vi "delete_element(array).vi"(8 "error in (no error)":errorcluster, 11 "data store (in)":cluster{"name":string, "address":string}[](array[cluster])) -> (0 "error out":errorcluster, 1 "deleted element":cluster{"name":string, "address":string}, 2 "element found ?":bool, 3 "data store (out)":cluster{"name":string, "address":string}[](array[cluster]))   [LabVIEW 2018]
panel:
  in  "name":string
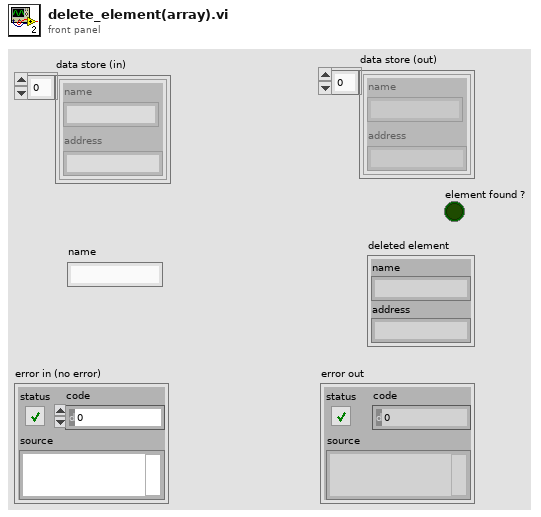
[diagram p1: front panel]
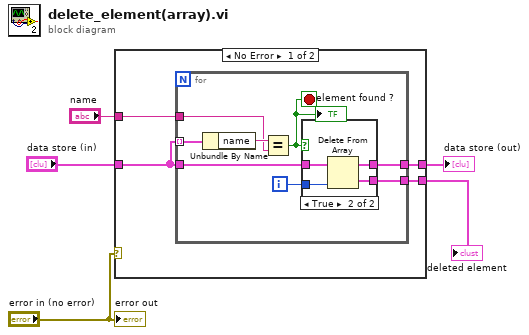
[diagram p0: block diagram]
diagram:
  n1 = case shown="No Error" "error in (no error)" {
    tunnel: "data store (in)" -> [w8 w23]
    tunnel: "name" -> [w9 _]
    tunnel: [w7 w23] -> w2
    tunnel: [w6 _] -> w1
    frame No Error {
      n2 = for {
        tunnel: w8 -> [w17] mode=indexing
        tunnel: w9 -> [w15]
        tunnel: w8 -> [w13]
        tunnel: [w12] -> w7
        tunnel: [w10] -> w6
        i -> [w14]
        stop <- w11 stop-if-true
        n3 = Unbundle By Name(w17) -> ("name"=w16:string)
        n4 = Equal?(x=w16, y=w15) -> (x = y?=w11:bool)
        "element found ?" <- w11
        n5 = case shown="True" w11 {
          tunnel: w14 -> [_ w22]
          tunnel: w13 -> [w18 w21]
          tunnel: [w18 w20] -> w12
          tunnel: [_ w19] -> w10
          frame False {
          }
          frame True {
            n6 = Delete From Array(array=w21, index=w22) -> (deleted portion=w19:cluster{"name":string, "address":string}, array with subset deleted=w20:cluster{"name":string, "address":string}[])  [unwired: 1 in]
          }
        }
      }
    }
    frame Error {
    }
  }
  "data store (out)" <- w2
  "deleted element" <- w1
  "error out" <- "error in (no error)"
